vi "lab1_commlab_is_fun.vi"() -> ()   [LabVIEW 2014]
panel:
  in  "expected result":string="001000010110111001110101011001100010000001110011011010010010000001100010011000010110110001101101011011010110111101000011000000000000000000000000000000000000000000001111000000000000111111000110101010101001001100001111"
  out "Result":string
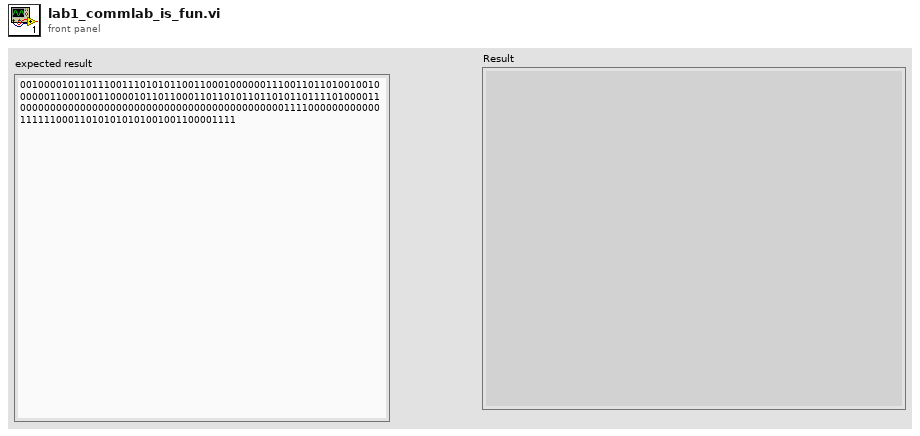
[diagram p1: front panel]
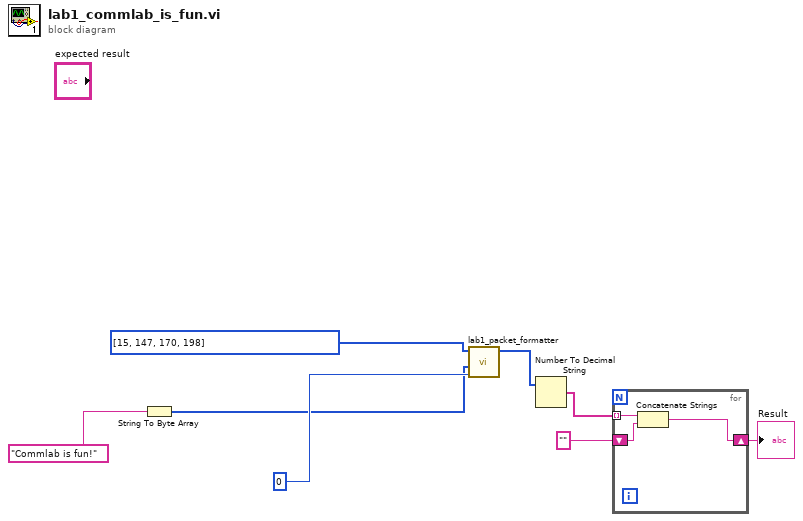
[diagram p0: block diagram]
diagram:
  n1 = String To Byte Array(string="Commlab is fun!" ("String")) -> (unsigned byte array=w5:u8[])
  n2 = call "lab1_packet_formatter.vi"("counter"=0, "payload(bytes array)"=w5, "preamble(bytes array)"=u8[] [15, 147, 170, 198] ("Array")) -> ("bitstream"=w4:i16[])  [unwired: 8 in]
  n3 = Number To Decimal String(number=w4) -> (decimal integer string=w2:string[])  [unwired: 1 in]
  n4 = for {
    shift-right: [w9] -> w1
    shift-left: "" -> [w11]
    tunnel: w2 -> [w10] mode=indexing
    n5 = Concatenate Strings(w10, w11) -> (w9:string)
  }
  "Result" <- w1
